vi "Adjust Splitter.vi"(8 "error in":errorcluster, 9 "Show":bool, 10 "Splitter Info":T1, 11 "Report Viewer in":refnum<class "Report Viewer.lvclass">) -> (0 "error out":errorcluster, 3 "Report Viewer out":refnum<class "Report Viewer.lvclass">)   [LabVIEW 2023, in "Report Viewer.lvlib" / "Report Viewer.lvclass"]
doc: "This override is here so child classes can act on a show/hide event.\nPrime panel does not adjust splitters"
uses:
  Library/Report Viewer.lvclass
  builds/Base Software/Panels/Prime Panel.lvlibp/Project/Prime Panel.lvclass
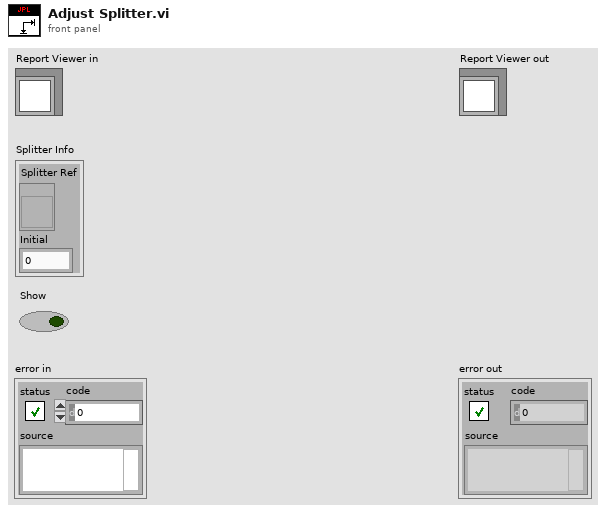
[diagram p1: front panel]
types:
  T1 = cluster{"Splitter Ref":refnum<vi>, "Initial":i32}
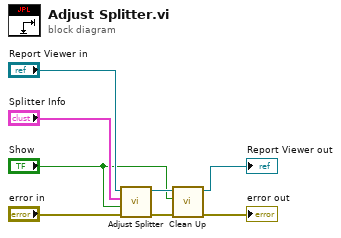
[diagram p0: block diagram]
diagram:
  n1 = call-parent "Adjust Splitter.vi"("error in"="error in", "Show"="Show", "Splitter Info"="Splitter Info", "Prime Panel in"="Report Viewer in") -> ("error out"=w4:errorcluster, "Prime Panel out"=w5:refnum<class "Report Viewer.lvclass">)  [unwired: 6 in]
  n2 = call "Clean Up.vi"("error in"=w4, "Show"="Show", "Report Viewer in"=w5) -> ("error out"=→"error out":errorcluster, "Report Viewer out"=→"Report Viewer out":refnum<class "Report Viewer.lvclass">)  [unwired: 7 in]
